vi "Publish Counter.vi"(8 "error in":errorcluster, 10 "Counter Data":dbl[](array[numeric]), 11 "BNT_DAQmx-MCSV in":refnum<class "BNT_DAQmx-MCSV.lvclass">) -> (0 "error out":errorcluster, 3 "BNT_DAQmx-MCSV out":refnum<class "BNT_DAQmx-MCSV.lvclass">)   [LabVIEW 2021, in "BNT_DAQmx.lvlib" / "BNT_DAQmx-MCSV.lvclass"]
doc: "Publish counter values if changed."
uses:
  BNT_DAQmx-MCSV.lvclass
  BNT_DAQmx-MCSV.lvclass/BNT_DAQmx-MCSV.ctl
  CSPP_Core/Classes/CSPP_ProcessVariables/PVConnection/PVConnection.lvclass/PVConnection.ctl
  CSPP_Core/Classes/CSPP_ProcessVariables/ProcessVariable/PV.lvclass/PV.ctl
  CSPP_Core/Classes/CSPP_ProcessVariables/ProcessVariable/Write Data.vi
  CSPP_Core/Classes/CSPP_ProcessVariables/ProcessVariable/Write Error.vi
  CSPP_Core/Classes/CSPP_ProcessVariables/ProcessVariable/Write Quality.vi
  CSPP_Core/Classes/CSPP_ProcessVariables/ProcessVariable/Write status.vi
  CSPP_Core/Classes/CSPP_ProcessVariables/ProcessVariable/Write Timestamp.vi
  CSPP_Core/Classes/CSPP_ProcessVariables/ProcessVariable/PV.lvclass
  CSPP_Core/Classes/CSPP_ProcessVariables/PVConnection/PVConnection.lvclass
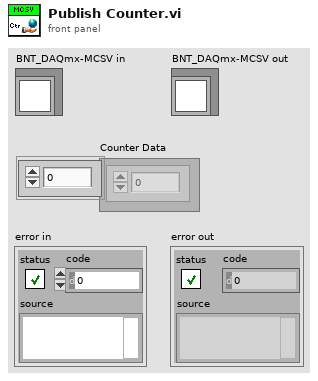
[diagram p1: front panel]
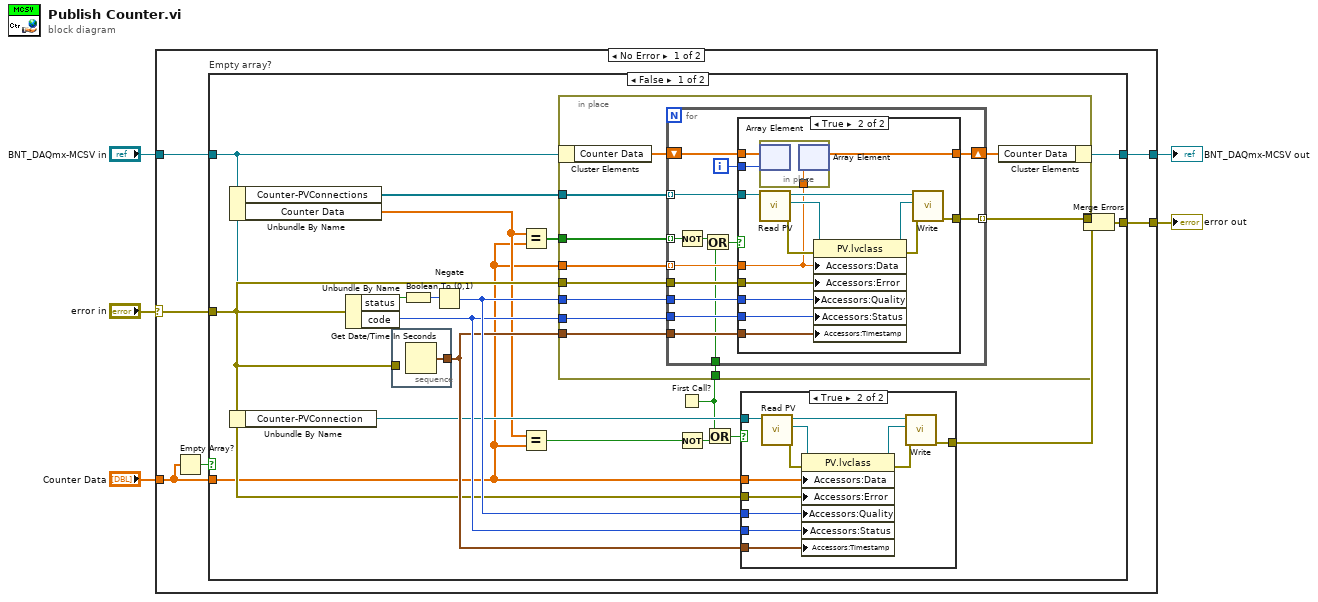
[diagram p0: block diagram]
diagram:
  n1 = case shown="No Error" "error in" {
    selector: "error in" -> [w11 w92]
    tunnel: [w10 w92] -> w4
    tunnel: [w8 w91] -> w2
    tunnel: "BNT_DAQmx-MCSV in" -> [w9 w91]
    tunnel: "Counter Data" -> [w6 _]
    frame No Error {
      n2 = Empty Array?(array=w6) -> (empty?=w7:bool)
      n3 = case "Empty array?" shown="False" w7 {
        tunnel: w11 -> [w24 w89]
        tunnel: [w22 w89] -> w10
        tunnel: w6 -> [w14 _]
        tunnel: w9 -> [w18 w90]
        tunnel: [w17 w90] -> w8
        frame False {
          n4 = Unbundle By Name(w18) -> ("Counter-PVConnections"=w23:refnum<class "PVConnection.lvclass">[], "Counter Data"=w19:dbl[])
          n5 = Unbundle By Name(w18) -> ("Counter-PVConnection"=w21:refnum<class "PVConnection.lvclass">)
          n6 = Unbundle By Name(w24) -> ("status"=w30:bool, "code"=w27:i32)
          n7 = stacked-sequence {
            tunnel: [w32] -> w26
            tunnel: w24 -> [_]
            frame #0 {
              n8 = Get Date/Time In Seconds() -> (seconds since 1Jan1904=w32:timestamp)
            }
          }
          n9 = Boolean To (0,1)(Boolean=w30) -> (0, 1=w29:i16)
          n10 = Negate(x=w29) -> (-x=w28:i16)
          n11 = Equal?(x=w19, y=w14) -> (x = y?=w20:bool[])
          n12 = Equal?(x=w19, y=w14) -> (x = y?=w16:bool)
          n13 = First Call?() -> (First Call?: T/F=w13:bool)
          n14 = in-place {
            in-place-border: [w43] -> w31
            in-place-border: w28 -> [w42]
            in-place-border: w27 -> [w41]
            in-place-border: w26 -> [w40]
            in-place-border: w24 -> [w39]
            in-place-border: w23 -> [w38]
            in-place-border: w14 -> [w37]
            in-place-border: w20 -> [w36]
            in-place-border: w13 -> [w33]
            n15 = in-place-cluster #1(w18) -> ("Counter Data"=w35:dbl[])
            n16 = for {
              tunnel: w38 -> [w51] mode=indexing
              tunnel: w37 -> [w57] mode=indexing
              tunnel: w39 -> [w56]
              tunnel: [w55] -> w43 mode=indexing
              tunnel: w42 -> [w54]
              tunnel: w41 -> [w53]
              tunnel: w40 -> [w52]
              tunnel: w36 -> [w50] mode=indexing
              shift-right: [w47] -> w34
              shift-left: w35 -> [w48]
              tunnel: w33 -> [w45]
              i -> [w49]
              n17 = Not(x=w50) -> (.not. x?=w44:bool)
              n18 = Or(x=w44, y=w45) -> (x .or. y?=w46:bool)
              n19 = case shown="True" w46 {
                tunnel: w57 -> [_ w61]
                tunnel: w56 -> [w59 w74]
                tunnel: [w59 w71] -> w55
                tunnel: w54 -> [_ w70]
                tunnel: w53 -> [_ w69]
                tunnel: w52 -> [_ w68]
                tunnel: w51 -> [_ w67]
                tunnel: w49 -> [_ w63]
                tunnel: w48 -> [w58 w62]
                tunnel: [w58 w60] -> w47
                frame False {
                }
                frame True {
                  n20 = in-place {
                    in-place-border: w61 -> [w75]
                    n21 = in-place-array #2(w62, w63) -> ()  [unwired: 1 out]
                    n22 = in-place-array #2(w75) -> (w60:dbl[])  [unwired: 1 out]
                  }
                  n23 = call "Read PV.vi"("PVConnection in"=w67) -> ("error out"=w64:errorcluster, "PV"=w65:refnum<class "PV.lvclass">, "PVConnection out"=w66:refnum<class "PVConnection.lvclass">)  [unwired: 8 in]
                  n24 = property class="PV.lvclass"(reference=w65, error in=w64, "Accessors:Data"=w61, "Accessors:Error"=w74, "Accessors:Quality"=w70, "Accessors:Status"=w69, "Accessors:Timestamp"=w68) -> (reference out=w73:refnum<class "PV.lvclass">, error out=w72:errorcluster)
                  n25 = call "Write.vi"("error in (no error)"=w72, "PV"=w73, "PVConnection in"=w66) -> ("error out"=w71:errorcluster)  [unwired: 6 in, 2 out]
                }
              }
            }
            n26 = in-place-cluster #1("Counter Data"=w34) -> (w17:refnum<class "BNT_DAQmx-MCSV.lvclass">)
          }
          n27 = Not(x=w16) -> (.not. x?=w12:bool)
          n28 = Or(x=w13, y=w12) -> (x .or. y?=w15:bool)
          n29 = case shown="True" w15 {
            tunnel: w28 -> [_ w83]
            tunnel: w27 -> [_ w82]
            tunnel: w26 -> [_ w81]
            tunnel: [w76 w80] -> w25
            tunnel: w24 -> [w76 w79]
            tunnel: w21 -> [_ w78]
            tunnel: w14 -> [_ w77]
            frame False {
            }
            frame True {
              n30 = call "Read PV.vi"("PVConnection in"=w78) -> ("error out"=w84:errorcluster, "PV"=w85:refnum<class "PV.lvclass">, "PVConnection out"=w86:refnum<class "PVConnection.lvclass">)  [unwired: 8 in]
              n31 = property class="PV.lvclass"(reference=w85, error in=w84, "Accessors:Data"=w77, "Accessors:Error"=w79, "Accessors:Quality"=w83, "Accessors:Status"=w82, "Accessors:Timestamp"=w81) -> (reference out=w88:refnum<class "PV.lvclass">, error out=w87:errorcluster)
              n32 = call "Write.vi"("error in (no error)"=w87, "PV"=w88, "PVConnection in"=w86) -> ("error out"=w80:errorcluster)  [unwired: 6 in, 2 out]
            }
          }
          n33 = Merge Errors(w31, w25) -> (w22:errorcluster)
        }
        frame True {
        }
      }
    }
    frame Error {
    }
  }
  "error out" <- w4
  "BNT_DAQmx-MCSV out" <- w2
